vi "Get Available Objects for PDO.vi"(8 "error in":errorcluster, 11 "EDS in":refnum<class "EDS.lvclass">) -> (0 "error out":errorcluster, 2 "Entries":refnum<class "OD Entry.lvclass">[](array[class]), 3 "EDS out":refnum<class "EDS.lvclass">)   [LabVIEW 2024, in "EDS.lvclass"]
uses:
  EDS.lvclass
  OD Entry/OD Entry.lvclass
  EDS.lvclass/EDS.ctl
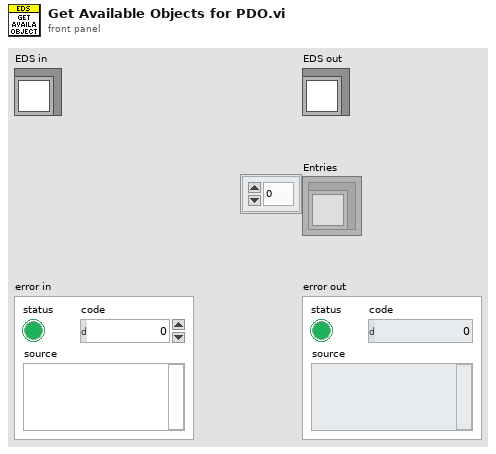
[diagram p1: front panel]
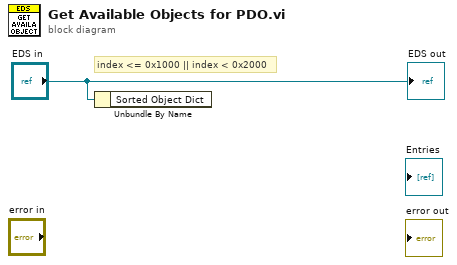
[diagram p0: block diagram]
diagram:
  # "index <= 0x1000 || index < 0x2000"
  n1 = Unbundle By Name("EDS in") -> ()  [unwired: 1 out]
  "EDS out" <- "EDS in"
